vi "Write String Register.vi"(7 "PDU Address String Params":T1 items=["Fluid name"=33160, "Capacity unit"=33272, "User tag"=61744], 8 "error in":errorcluster, 10 "String":string, 11 "MB_TCP session in":refnum<class "MB_Master_TCP.lvclass">) -> (0 "error out":errorcluster, 3 "MB session out":refnum<class "MB_Master_TCP.lvclass">)   [LabVIEW 2024, in "Bronkhorst Flexi-Flow ModbusTCP API.lvlib"]
uses:
  Bronkhorst Flexi-Flow ModbusTCP API.lvlib
  <vilib>/Plasmionique/MB Master/MB_Master_TCP/MB_Master_TCP.lvclass
  C:/Program Files/National Instruments/LabVIEW 2025/vi.lib/Plasmionique/MB Master/MB_Master/MB_Master.lvclass
  PDU Address String Params--ring.ctl
  <vilib>/Plasmionique/MB Master/MB Master.lvlib
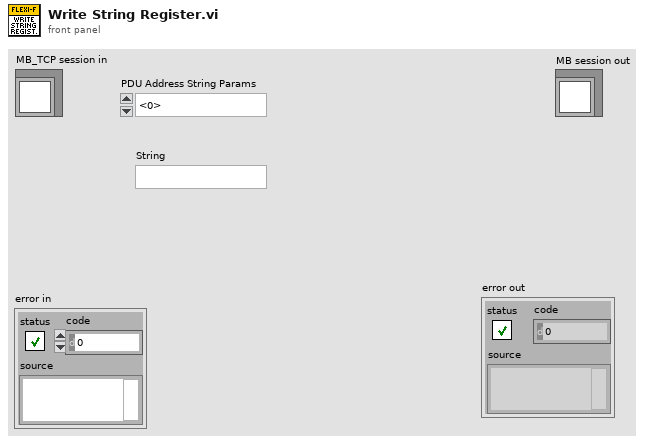
[diagram p1: front panel]
types:
  T1 = typedef "Bronkhorst Flexi-Flow ModbusTCP API.lvlib/PDU Address String Params--ring.ctl" = u16
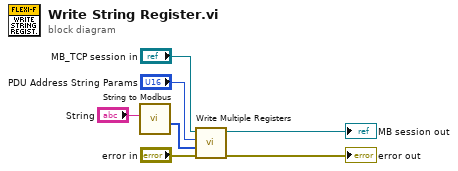
[diagram p0: block diagram]
diagram:
  n1 = call "String to Modbus.vi"("String"="String") -> ("Array"=w1:u16[])  [unwired: 10 in]
  n2 = call <vilib>:"Write Multiple Registers.vi"("error in (no error)"="error in", "values"=w1, "starting address"="PDU Address String Params", "MB session in"="MB_TCP session in") -> ("error out"=→"error out":errorcluster, "MB session out"=→"MB session out":refnum<class "MB_Master_TCP.lvclass">)  [unwired: 6 in]
